vi "Save_Raw_data.vi"(0 "PDLSTS":refnum<k24>, 1 "chk2scan":bool, 2 "exist_flag":bool, 3 "first_rangeflag":bool, 5 "Meas_monitor_struct":refnum<k24>[](array[refnum]), 9 "Data_struct":refnum<k24>[](array[refnum]), 11 "错误输入（无错误）":errorcluster, 12 "Meas_rang":i32[](array[numeric]), 14 "rangenumber":i32) -> (15 "错误输出":errorcluster)   [LabVIEW 2017]
doc: "Save mesurement raw data"
uses:
  D:/test/PDLSTS/LV_PDL_Sample/DLL/STSProcess.dll
  DLL/STSProcess.dll
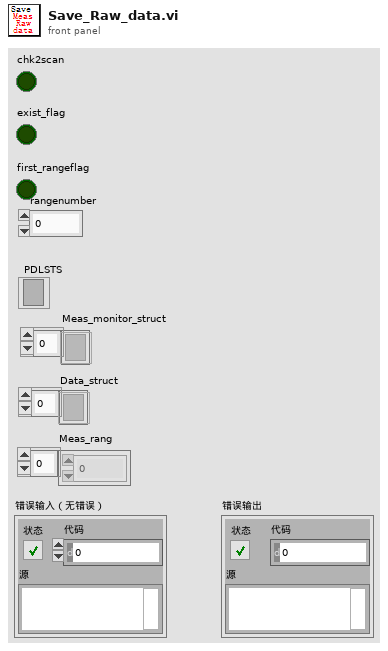
[diagram p1: front panel]
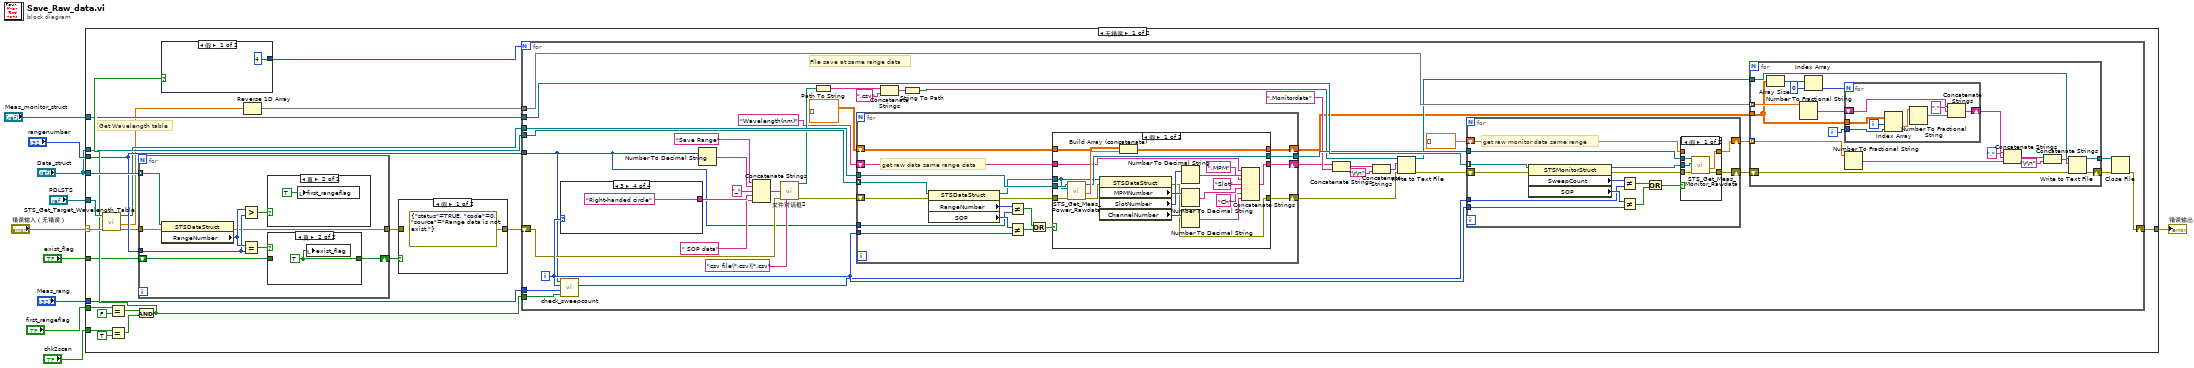
[diagram p0: block diagram]
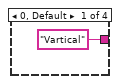
[diagram p4: hidden frame]
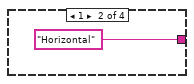
[diagram p5: hidden frame]
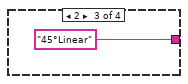
[diagram p6: hidden frame]
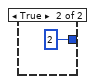
[diagram p7: hidden frame]
diagram:
  n1 = case shown="无错误" "错误输入（无错误）" {
    selector: "错误输入（无错误）" -> [w33 w186]
    tunnel: [w18 w186] -> w10
    tunnel: "PDLSTS" -> [w34 _]
    tunnel: "Data_struct" -> [w32 _]
    tunnel: "Meas_rang" -> [w23 _]
    tunnel: "rangenumber" -> [w22 _]
    tunnel: "chk2scan" -> [w28 _]
    tunnel: "Data_struct" -> [w21 _]
    tunnel: "Meas_monitor_struct" -> [w19 _]
    tunnel: "exist_flag" -> [w12 _]
    tunnel: "first_rangeflag" -> [w13 _]
    frame No Error {
      # "Get Wavelength table"
      n2 = call "STS_Get_Target_Wavelength_Table.vi"("错误输入（无错误）"=w33, ".NET引用句柄输入"=w34) -> ("error out"=w16:errorcluster, "wavelengths"=w15:dbl[], "引用输出"=w20:refnum<k24>)  [unwired: 7 in]
      n3 = Equal?(x=w13, y=FALSE) -> (x = y?=w26:bool)
      n4 = Equal?(x=w28, y=TRUE) -> (x = y?=w27:bool)
      n5 = And(x=w26, y=w27) -> (x .and. y?=w24:bool)
      n6 = for {
        tunnel: w32 -> [w182] mode=indexing
        tunnel: w22 -> [w179]
        tunnel: w16 -> [w177]
        tunnel: [w176] -> w31
        shift-right: [w175] -> w11
        shift-left: w12 -> [w174]
        n7 = property on="属性节点" class="STSDataStruct"(reference=w182, error in=w177) -> (error out=w176:errorcluster, "RangeNumber"=w180:i32)  [unwired: 1 out]
        n8 = Greater?(x=w180, y=w179) -> (0:w181:bool)
        n9 = Equal?(x=w180, y=w179) -> (x = y?=w178:bool)
        n10 = case shown="真" w181 {
          frame False {
          }
          frame True {
            n11 = local write "first_rangeflag"(TRUE ("first_rangeflag")) -> ()
          }
        }
        n12 = case shown="真" w178 {
          tunnel: [w183 w184] -> w175
          tunnel: w174 -> [w183 _]
          frame False {
          }
          frame True {
            w184 = TRUE ("exist_flag")
            n13 = local write "exist_flag"(w184) -> ()
          }
        }
      }
      n14 = case shown="假" w24 {
        tunnel: [4 2] -> w25
        frame False {
        }
        frame True {
        }
      }
      n15 = Reverse 1D Array(array=w15) -> (reversed array=w14:dbl[])
      n16 = case shown="假" w11 {
        tunnel: w31 -> [_ w173]
        tunnel: [errorcluster {"status"=TRUE, "code"=0, "source"="Range data is not exist."} ("error out") w173] -> w17
        frame False {
        }
        frame True {
        }
      }
      n17 = for {
        N: w25 -> [_]
        tunnel: w24 -> [w75]
        tunnel: w23 -> [w74]
        tunnel: w22 -> [w35]
        tunnel: w21 -> [w73]
        tunnel: w20 -> [w72]
        tunnel: w19 -> [w71]
        tunnel: w14 -> [w70]
        shift-right: [w67] -> w18
        shift-left: w17 -> [w66]
        i -> [w68]
        # "File save at same range data"
        n18 = case shown="3" w68 {
          tunnel: ["Vartical" "Horizontal" "45°Linear" "Right-handed circle"] -> w69
          frame 0, Default {
          }
          frame 1 {
          }
          frame 2 {
          }
          frame 3 {
          }
        }
        n19 = call "check_sweepcount.vi"("rangenumber"=w35, "sopcount"=w68, "Meas_rang"=w74, "chk2scan"=w75) -> ("sweepcount"=w65:i32)  [unwired: 6 in]
        n20 = Number To Decimal String(number=w35) -> (decimal integer string=w62:string)  [unwired: 1 in]
        n21 = Concatenate Strings("Save Range" ("字符串"), w62, "_" ("字符串"), w69, " SOP data" ("字符串")) -> (w58:string)
        n22 = call "文件对话框2"("default name"=w58, "error in"=w66, "pattern (all files)"="csv file(*.csv)|*.csv") -> ("selected path"=w54:path, "error out"=w43:errorcluster)  [unwired: 9 in, 2 out]
        n23 = Path To String(path=w54) -> (string=w55:string)
        n24 = for {
          tunnel: w73 -> [w141] mode=indexing
          tunnel: w35 -> [w126]
          tunnel: w72 -> [w137]
          shift-right: [w133] -> w40
          shift-left: w43 -> [w139]
          shift-right: [w134] -> w46
          shift-left: sgl[][] [] -> [w135]
          tunnel: [w132] -> w64
          tunnel: w68 -> [w130]
          shift-right: [w124] -> w41
          shift-left: "Wavelength(nm)" -> [w125]
          # "get raw data same range data"
          n25 = property on="属性节点" class="STSDataStruct"(reference=w141, error in=w139) -> (reference out=w136:refnum<k24>, error out=w138:errorcluster, "RangeNumber"=w140:i32, "SOP"=w131:i32)
          n26 = Not Equal?(x=w140, y=w126) -> (x != y?=w129:bool)
          n27 = Not Equal?(x=w131, y=w130) -> (x != y?=w128:bool)
          n28 = Or(x=w129, y=w128) -> (x .or. y?=w127:bool)
          n29 = case shown="假" w127 {
            tunnel: w138 -> [w161 w164]
            tunnel: w137 -> [w160 w163]
            tunnel: w136 -> [w150 _]
            tunnel: w135 -> [w158 w165]
            tunnel: [w157 w165] -> w134
            tunnel: [w148 w164] -> w133
            tunnel: [w156 w163] -> w132
            tunnel: w125 -> [w152 w162]
            tunnel: [w151 w162] -> w124
            frame False {
              n30 = call "STS_Get_Meas_Power_Rawdata.vi"("错误输入（无错误）"=w161, "setting"=w150, ".NET引用句柄输入"=w160) -> ("error out"=w149:errorcluster, "powerdata"=w159:sgl[], "引用输出"=w156:refnum<k24>)  [unwired: 6 in]
              n31 = property on="属性节点" class="STSDataStruct"(reference=w150, error in=w149) -> (error out=w148:errorcluster, "MPMNumber"=w153:i32, "SlotNumber"=w154:i32, "ChannelNumber"=w155:i32)  [unwired: 1 out]
              n32 = Build Array (concatenate)(w158, w159) -> (w157:sgl[][])
              n33 = Number To Decimal String(number=w153) -> (decimal integer string=w146:string)  [unwired: 1 in]
              n34 = Number To Decimal String(number=w154) -> (decimal integer string=w144:string)  [unwired: 1 in]
              n35 = Number To Decimal String(number=w155) -> (decimal integer string=w142:string)  [unwired: 1 in]
              n36 = Concatenate Strings(w152, ",MPM" ("字符串"), w146, "Slot" ("字符串"), w144, "Ch" ("字符串"), w142) -> (w151:string)
            }
            frame True {
            }
          }
        }
        n37 = Concatenate Strings(w55, ".csv" ("名称或相对路径")) -> (w56:string)
        n38 = String To Path(string=w56) -> (path=w49:path)
        n39 = Concatenate Strings(w41, ",Monitordata" ("字符串")) -> (w50:string)
        n40 = Concatenate Strings(w50, "\r\n") -> (w52:string)
        n41 = Write to Text File(file (use dialog)=w49, text=w52, error in=w40) -> (refnum out=w48:refnum<file>, error out=w39:errorcluster)  [unwired: 1 in, 1 out]
        n42 = for {
          tunnel: w71 -> [w116] mode=indexing
          shift-right: [w110] -> w38
          shift-left: w39 -> [w115]
          tunnel: w64 -> [w111]
          shift-right: [w109] -> w45
          shift-left: sgl[] [] ("monitordata") -> [w108]
          tunnel: w68 -> [w103]
          tunnel: w65 -> [w102]
          # "get raw monitor data same range"
          n43 = property on="属性节点" class="STSMonitorStruct"(reference=w116, error in=w115) -> (reference out=w113:refnum<k24>, error out=w112:errorcluster, "SweepCount"=w114:i32, "SOP"=w107:i32)
          n44 = Not Equal?(x=w114, y=w102) -> (x != y?=w105:bool)
          n45 = Not Equal?(x=w107, y=w103) -> (x != y?=w106:bool)
          n46 = Or(x=w105, y=w106) -> (x .or. y?=w104:bool)
          n47 = case shown="假" w104 {
            tunnel: w113 -> [w121 _]
            tunnel: w112 -> [w120 w123]
            tunnel: w111 -> [w119 _]
            tunnel: [w118 w123] -> w110
            tunnel: [w117 w122] -> w109
            tunnel: w108 -> [_ w122]
            frame False {
              n48 = call "STS_Get_Meas_Monitor_Rawdata.vi"("错误输入（无错误）"=w120, "setting"=w121, ".NET引用句柄输入"=w119) -> ("error out"=w118:errorcluster, "monitordata"=w117:sgl[])  [unwired: 6 in, 1 out]
            }
            frame True {
            }
          }
        }
        n49 = for {
          tunnel: w70 -> [w93] mode=indexing
          tunnel: w48 -> [w85]
          tunnel: [w84] -> w37
          shift-right: [w90] -> w36
          shift-left: w38 -> [w91]
          tunnel: w46 -> [w81]
          tunnel: w45 -> [w80] mode=indexing
          i -> [w82]
          n50 = Array Size(array=w81) -> (size(s)=w88:i32[])
          n51 = Number To Fractional String(number=w93) -> (F-format string=w92:string)  [unwired: 3 in]
          n52 = Index Array(array=w88, index=0 ("索引")) -> (element=w86:i32)
          n53 = for {
            N: w86 -> [_]
            tunnel: w81 -> [w101]
            tunnel: w82 -> [w100]
            shift-right: [w96] -> w77
            shift-left: w92 -> [w97]
            i -> [w99]
            n54 = Index Array(array=w101, index (row)=w99, index (col)=w100) -> (element=w98:sgl)
            n55 = Number To Fractional String(number=w98) -> (F-format string=w94:string)  [unwired: 3 in]
            n56 = Concatenate Strings(w97, "," ("字符串"), w94) -> (w96:string)
          }
          n57 = Number To Fractional String(number=w80) -> (F-format string=w79:string)  [unwired: 3 in]
          n58 = Concatenate Strings(w77, "," ("字符串"), w79) -> (w76:string)
          n59 = Concatenate Strings(w76, "\r\n") -> (w89:string)
          n60 = Write to Text File(file (use dialog)=w85, text=w89, error in=w91) -> (refnum out=w84:refnum<file>, error out=w90:errorcluster)  [unwired: 1 in, 1 out]
        }
        n61 = Close File(refnum=w37, error in=w36) -> (error out=w67:errorcluster)  [unwired: 1 out]
      }
    }
    frame Error {
    }
  }
  "错误输出" <- w10
